vi "Open File.vi"(8 "error in (no error)":errorcluster, 10 "Path":path, 11 "ROFile in":refnum<class "ROFile.lvclass">) -> (0 "error out":errorcluster, 3 "ROFile out":refnum<class "ROFile.lvclass">)   [LabVIEW 2021, in "ROFile.lvclass"]
uses:
  ROFile.lvclass
  E:/Programs/LabVIEW/Other Stuff/GLA Summit 2025/LVClassyFile/1. Using Classes/Classes/File/File.lvclass
  File/File.lvclass/File.ctl
  File/File.lvclass
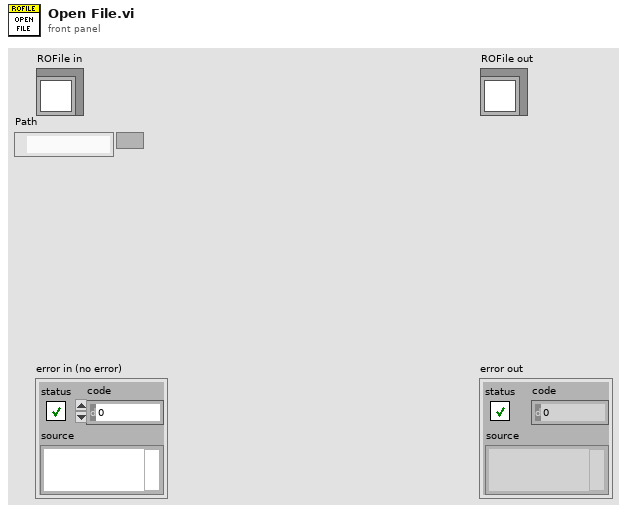
[diagram p1: front panel]
types:
  T1 = enum16{"open", "replace", "create", "open or create", "replace or create", "replace or create with confirmation"}
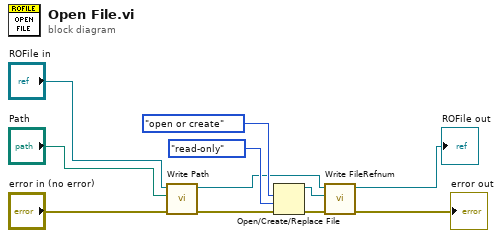
[diagram p0: block diagram]
diagram:
  n1 = call "Write Path.vi"("error in (no error)"="error in (no error)", "Path"="Path", "File in"="ROFile in") -> ("error out"=w10:errorcluster, "File out"=w3:refnum<class "ROFile.lvclass">)  [unwired: 7 in]
  n2 = Open/Create/Replace File(error in=w10, operation (0:open)=T1."open or create", access (0:read/write)=enum16{"read/write", "read-only", "write-only"}."read-only") -> (refnum out=w1:refnum<file>, error out=w7:errorcluster)  [unwired: 3 in, 1 out]
  n3 = call "Write FileRefnum.vi"("error in (no error)"=w7, "FileRefnum"=w1, "File in"=w3) -> ("error out"=→"error out":errorcluster, "File out"=→"ROFile out":refnum<class "ROFile.lvclass">)  [unwired: 7 in]
